vi "test_Multiple Static Single Channel Command-Response Messages using Trigger with Protection.vi"(8 "error in (no error)":errorcluster, 11 "TestCase in":refnum<class "Instrument Addon Common System Tests.lvclass">) -> (0 "error out":errorcluster, 3 "TestCase out":refnum<class "Instrument Addon Common System Tests.lvclass">)   [LabVIEW 2018, in "Instrument Addon Common System Tests.lvclass"]
uses:
  Instrument Addon Common System Tests.lvclass
  C:/Users/nitest/Git/NI VS Test Utilities/VeriStandTestCase/VeriStandTestCase.lvclass
  <vilib>/addons/_JKI Toolkits/VI Tester/TestCase.llb/TestCase.lvclass
  C:/Program Files (x86)/National Instruments/LabVIEW 2018/vi.lib/addons/_JKI Toolkits/VI Tester/TestCase.llb/TestCase.lvclass
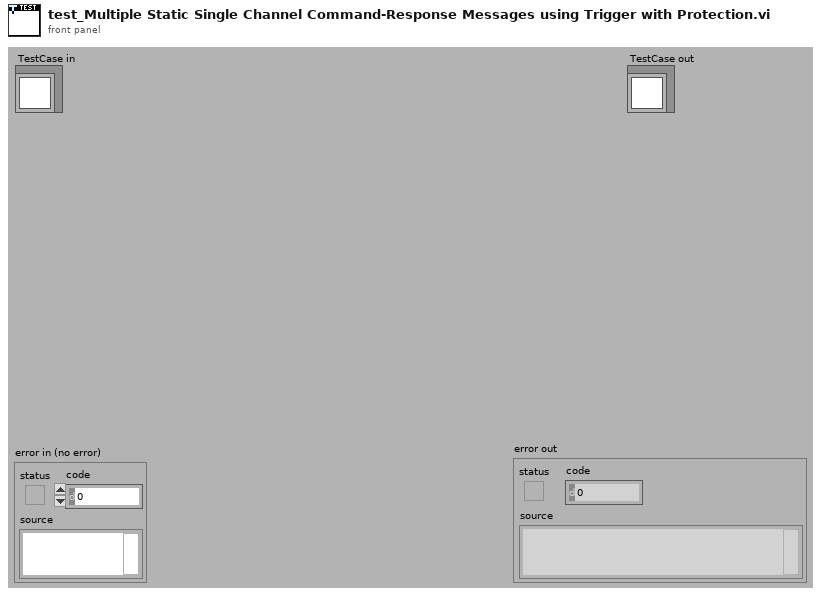
[diagram p1: front panel]
types:
  T1 = typedef "NI_VS Workspace ExecutionAPI.lvlib/WorkspaceAPI.ctl" = refnum<k24>
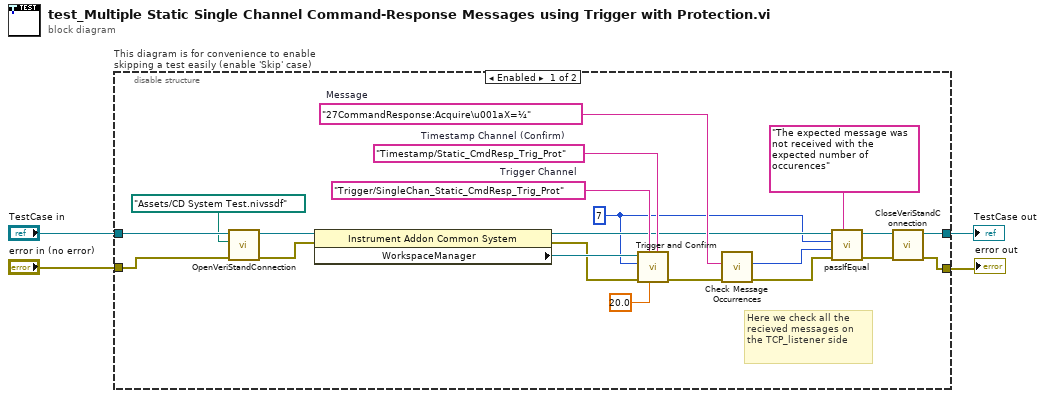
[diagram p0: block diagram]
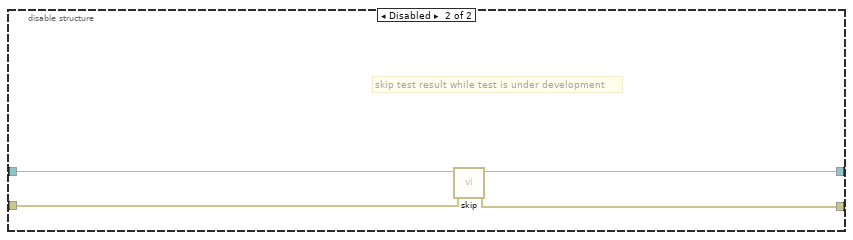
[diagram p2: hidden frame]
diagram:
  n1 = disable-structure "This diagram is for convenience to enable skipping a test easily (enable 'Skip' case)" shown="Enabled" {
    disable-tunnel: "TestCase in" -> [w23 w29]
    disable-tunnel: [w24 w27] -> w1
    disable-tunnel: [w25 w28] -> w3
    disable-tunnel: "error in (no error)" -> [w21 w26]
    frame Enabled {
      w7 = 7
      w16 = "Timestamp/Static_CmdResp_Trig_Prot"  # Timestamp Channel (Confirm)
      w12 = "27CommandResponse:Acquire\u001aX=¼"  # Message
      w17 = "Trigger/SingleChan_Static_CmdResp_Trig_Prot"  # Trigger Channel
      # "Here we check all the recieved messages on the TCP_listener side"
      n2 = call-dynamic "OpenVeriStandConnection.vi"("error in (no error)"=w21, "System Definition File"=path "Assets/CD System Test.nivssdf", "VeriStand Test Case in"=w23) -> ("error out"=w20:errorcluster, "VeriStand Test Case out"=w22:refnum<class "Instrument Addon Common System Tests.lvclass">)  [unwired: 6 in, 1 out]
      n3 = property class="Instrument Addon Common System "(reference=w22, error in=w20) -> (reference out=w10:refnum<class "Instrument Addon Common System Tests.lvclass">, error out=w15:errorcluster, "WorkspaceManager"=w18:T1)
      n4 = call "Trigger and Confirm.vi"("Timestamp Channel (Confirm)"=w16, "Timeout (s)"=20.0, "Trigger Channel"=w17, "error in (no error)"=w15, "Number of Triggers"=w7, "WorkspaceManager in"=w18) -> ("error out"=w14:errorcluster)  [unwired: 4 in, 1 out]
      n5 = call "Check Message Occurrences.vi"("error in (no error)"=w14, "Message"=w12) -> ("error IO"=w11:errorcluster, "Occurences"=w6:i32)  [unwired: 8 in]
      n6 = call-dynamic "passIfEqual.vi"("custom report message (\"\")"="The expected message was not received with the expected number of occurences" ("custom report message (\"\")"), "error in (no error)"=w11, "y"=w6, "x"=w7, "TestCase in"=w10) -> ("error out"=w8:errorcluster, "TestCase out"=w9:refnum<class "Instrument Addon Common System Tests.lvclass">)  [unwired: 5 in]
      n7 = call-dynamic "CloseVeriStandConnection.vi"("error in (no error)"=w8, "VeriStand Test Case in"=w9) -> ("error out"=w25:errorcluster, "VeriStand Test Case out"=w24:refnum<class "Instrument Addon Common System Tests.lvclass">)  [unwired: 8 in]
    }
    frame Disabled {
      # "skip test result while test is under development"
      n8 = call <vilib>:"skip.vi"("error in (no error)"=w26, "TestCase in"=w29) -> ("error out"=w28:errorcluster, "TestCase out"=w27:refnum<class "Instrument Addon Common System Tests.lvclass">)  [unwired: 8 in]
    }
  }
  "error out" <- w3
  "TestCase out" <- w1
